vi "BoxTempJT.vi"() -> (0 "Box Temperature":dbl format="%#_13g")   [LabVIEW 2016]
uses:
  Instrument_Setup.vi
  <vilib>/Instr/_visa.llb/VISA Configure Serial Port (Instr).vi
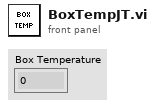
[diagram p1: front panel]
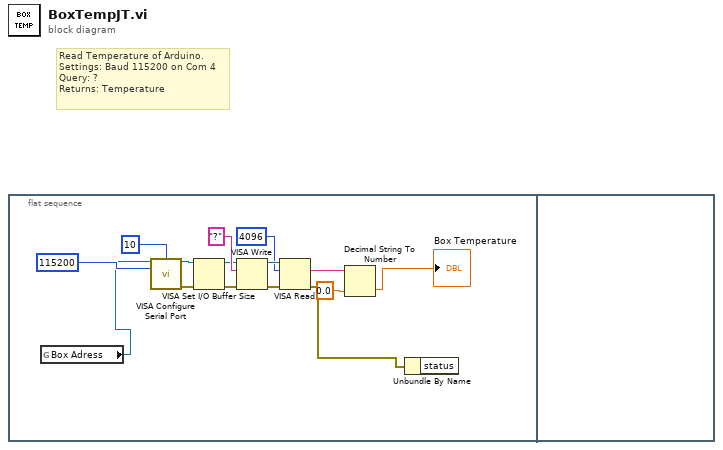
[diagram p0: block diagram]
diagram:
  # "Read Temperature of Arduino. \nSettings: Baud 115200 on Com 4\nQuery: ?\nReturns: Temperature"
  n1 = flat-sequence {
    frame #0 {
      n2 = global read "Instrument_Setup.vi" "Box Adress"() -> (w3:refnum<visa-resource-name>)
      n3 = call-poly "VISA Configure Serial Port"("VISA resource name"=w3, "termination char\n(0xA = '\\n' = LF)"=u8 10 ("termination char\n(0xA = '\\n' = LF)"), "baud rate (9600)"=115200) -> ("VISA resource name out"=w7:refnum<visa-resource-name>, "error out"=w9:errorcluster)  [unwired: 11 in]
      n4 = VISA Set I/O Buffer Size(VISA resource name=w7, error in (no error)=w9) -> (VISA resource name out=w8:refnum<visa-resource-name>, error out=w6:errorcluster)  [unwired: 2 in]
      n5 = VISA Write(VISA resource name=w8, write buffer="?", error in (no error)=w6) -> (VISA resource name out=w15:refnum<visa-resource-name>, error out=w14:errorcluster)  [unwired: 1 out]
      n6 = VISA Read(VISA resource name=w15, byte count=4096, error in (no error)=w14) -> (read buffer=w5:string, error out=w1:errorcluster)  [unwired: 2 out]
      n7 = Decimal String To Number(string=w5, default (0L)=0.0) -> (number=→"Box Temperature":dbl)  [unwired: 1 in, 1 out]
      n8 = Unbundle By Name(w1) -> ()  [unwired: 1 out]
    }
    frame #1 {
    }
  }
